vi "test_model.vi"() -> (3 "out":refnum<class "KernelRidge.lvclass">)   [LabVIEW 2020]
uses:
  Supervised/KernelRidge/KernelRidge.lvclass
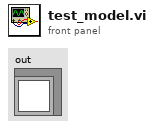
[diagram p1: front panel]
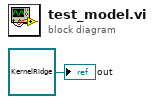
[diagram p0: block diagram]
diagram:
  "out" <- refnum<class "KernelRidge.lvclass"> refnum ("model")
